vi "Update GU Selection List.vi"(8 "error in":errorcluster, 10 "Curr Cal Cfg":T1, 11 "Ctrl Ref":T2) -> (0 "error out":errorcluster)   [LabVIEW 2020, in "GUCalibration2.lvlib"]
uses:
  GUCalibration2.lvlib
  Controls/GU Arrange UI Ref.ctl
  Controls/Config Data Type.ctl
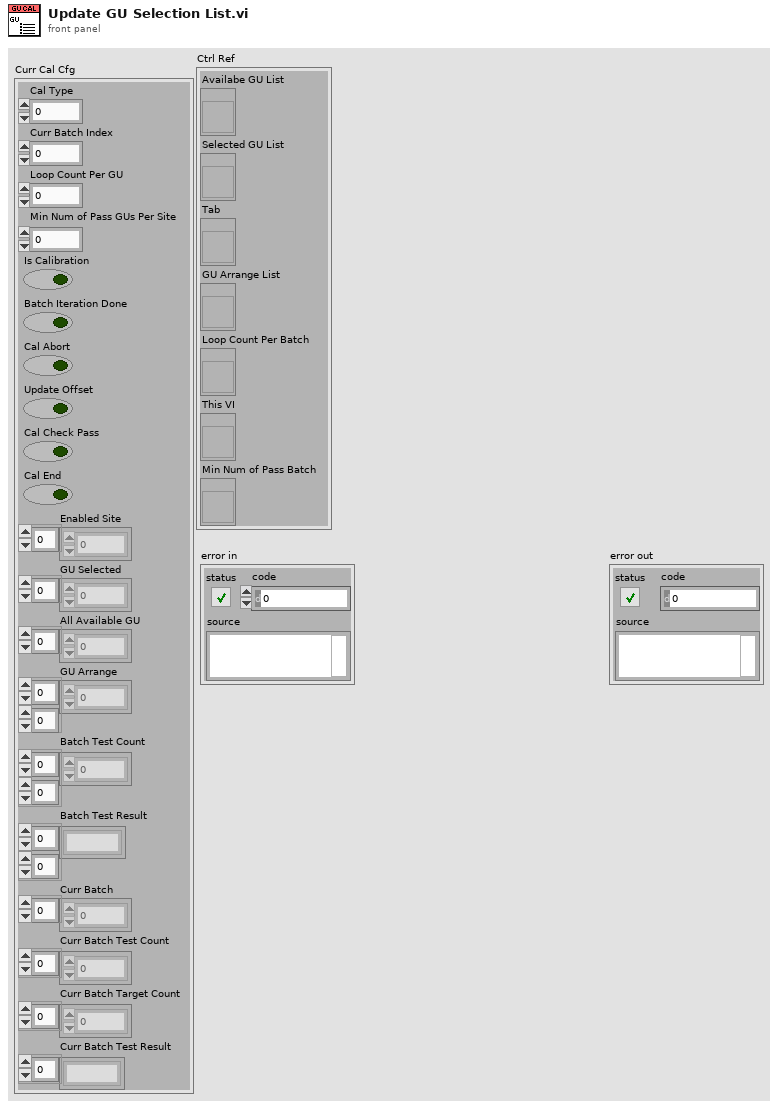
[diagram p1: front panel]
types:
  T1 = typedef "GUCalibration2.lvlib/Config Data Type.ctl" = cluster{"Cal Type":i32, "Curr Batch Index":i32, "Loop Count Per GU":i32, "Min Num of Pass GUs Per Site":i32, "Is Calibration":bool, "Batch Iteration Done":bool, "Cal Abort":bool, "Update Offset":bool, "Cal Check Pass":bool, "Cal End":bool, "Enabled Site":i32[], "GU Selected":i32[], "All Available GU":i32[], "GU Arrange":i32[][], "Batch Test Count":i32[][], "Batch Test Result":string[][], "Curr Batch":i32[], "Curr Batch Test Count":i32[], "Curr Batch Target Count":i32[], "Curr Batch Test Result":string[]}
  T2 = typedef "GUCalibration2.lvlib/GU Arrange UI Ref.ctl" = cluster{"Availabe GU List":refnum<vi>, "Selected GU List":refnum<vi>, "Tab":refnum<vi>, "GU Arrange List":refnum<vi>, "Loop Count Per Batch":refnum<vi>, "This VI":refnum<vi>, "Min Num of Pass Batch":refnum<vi>}
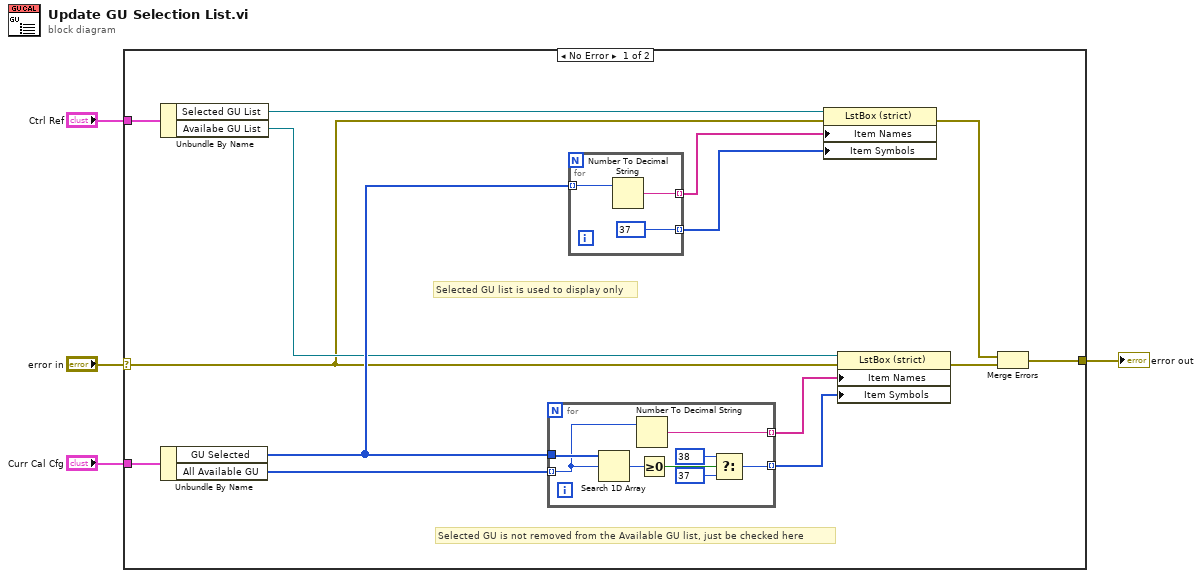
[diagram p0: block diagram]
diagram:
  n1 = case shown="No Error" "error in" {
    selector: "error in" -> [w5 w30]
    tunnel: "Ctrl Ref" -> [w18 _]
    tunnel: "Curr Cal Cfg" -> [w17 _]
    tunnel: [w8 w30] -> w2
    frame No Error {
      # "Selected GU is not removed from the Available GU list, just be checked here"
      # "Selected GU list is used to display only"
      n2 = Unbundle By Name(w18) -> ("Selected GU List"=w7:refnum<vi>, "Availabe GU List"=w6:refnum<vi>)
      n3 = Unbundle By Name(w17) -> ("GU Selected"=w11:i32[], "All Available GU"=w16:i32[])
      n4 = for {
        tunnel: w16 -> [w20] mode=indexing
        tunnel: w11 -> [w26]
        tunnel: [w21] -> w14 mode=indexing
        tunnel: [w19] -> w15 mode=indexing
        n5 = Search 1D Array(1D array=w26, element=w20) -> (index of element=w25:i32)  [unwired: 1 in]
        n6 = Number To Decimal String(number=w20) -> (decimal integer string=w19:string)  [unwired: 1 in]
        n7 = Greater Or Equal To 0?(x=w25) -> (x >= 0?=w24:bool)
        n8 = Select(t=38, s=w24, f=37) -> (s? t:f=w21:i32)
      }
      n9 = for {
        tunnel: w11 -> [w29] mode=indexing
        tunnel: [w28] -> w12 mode=indexing
        tunnel: [37] -> w13 mode=indexing
        n10 = Number To Decimal String(number=w29) -> (decimal integer string=w28:string)  [unwired: 1 in]
      }
      n11 = property class="LstBox (strict)"(reference=w7, error in=w5, "Item Names"=w12, "Item Symbols"=w13) -> (error out=w10:errorcluster)  [unwired: 1 out]
      n12 = property class="LstBox (strict)"(reference=w6, error in=w5, "Item Names"=w15, "Item Symbols"=w14) -> (error out=w9:errorcluster)  [unwired: 1 out]
      n13 = Merge Errors(w10, w9) -> (w8:errorcluster)
    }
    frame Error {
    }
  }
  "error out" <- w2
